vi "Score Particles.vi"(8 "Area Size Limit":i32=444, 9 "Particle Count Limit":i32=10, 11 "Image Refnum in":T1) -> (0 "Circle Info":cluster{dbl, dbl, dbl}[](array[cluster]), 2 "Scored Particle Info":T2(array[cluster]), 3 "Image Refnum out":T1)   [LabVIEW 2012]
doc: "Score the largest particles in the image to determine how well they match the target attributes. Specifically, calculate how rectangular a particle is, inspect its aspect ratio, and determine if it is hollow (having pixels on around the edges, but off in the large center)."
uses:
  <vilib>/vision/Image Controls.llb/IMAQ Image.ctl
  <vilib>/vision/NI_Vision_Development_Module.lvlib
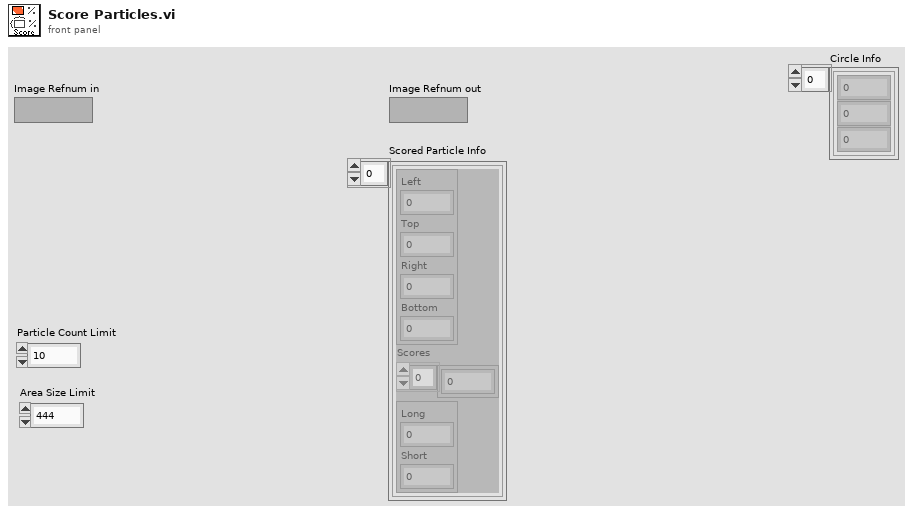
[diagram p1: front panel]
types:
  T1 = typedef "IMAQ Image.ctl" = refnum<image>
  T2 = cluster{cluster{"Left":dbl, "Top":dbl, "Right":dbl, "Bottom":dbl}, "Scores":dbl[], cluster{"Long":dbl, "Short":dbl}}[]
  T3 = typedef "Particle Parameters" = i32
  T4 = typedef "Image Type" = u32
  T5 = cluster{"Left":dbl, "Top":dbl, "Right":dbl, "Bottom":dbl}
  T6 = cluster{cluster{"Left":dbl, "Top":dbl, "Right":dbl, "Bottom":dbl}, dbl[], cluster{"Numeric":dbl, "Numeric":dbl}}
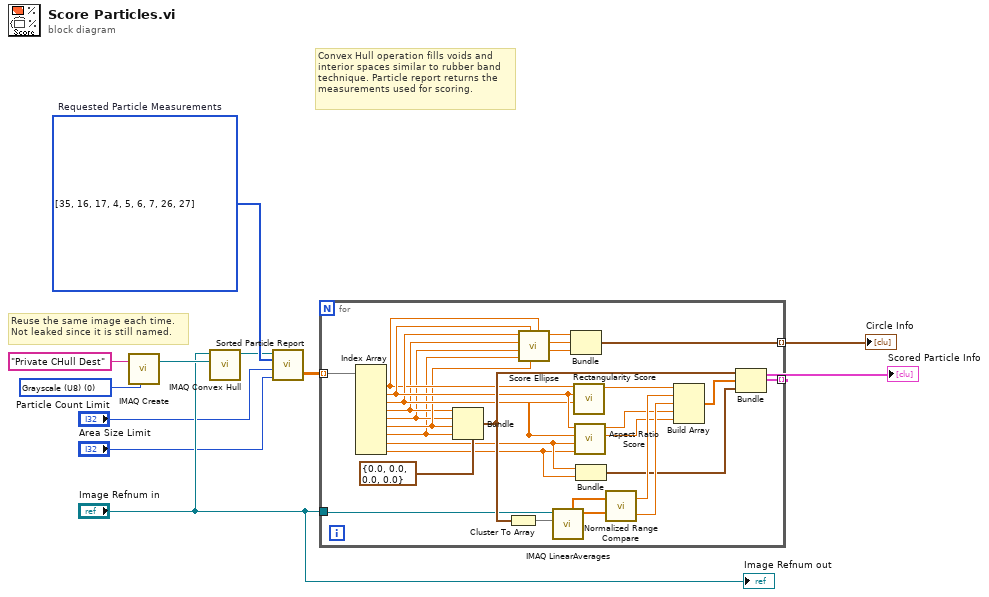
[diagram p0: block diagram]
diagram:
  w3 = T3[] [35, 16, 17, 4, 5, 6, 7, 26, 27] items=["Center of Mass X", "Center of Mass Y", "First Pixel X", "First Pixel Y", "Bounding Rect Left", "Bounding Rect Top", "Bounding Rect Right", "Bounding Rect Bottom", "Max Feret Diameter Start X", "Max Feret Diameter Start Y", "Max Feret Diameter End X", "Max Feret Diameter End Y", "Max Horiz. Segment Length Left", "Max Horiz. Segment Length Right", "Max Horiz. Segment Length Row", "-", "Bounding Rect Width", "Bounding Rect Height", "Bounding Rect Diagonal", "Perimeter", "Convex Hull Perimeter", "Holes' Perimeter", "Max Feret Diameter", "Equivalent Ellipse Major Axis", "Equivalent Ellipse Minor Axis", "Equivalent Ellipse Minor Axis (Feret)", "Equivalent Rect Long Side", "Equivalent Rect Short Side", "Equivalent Rect Diagonal", "Equivalent Rect Short Side (Feret)", "Average Horiz. Segment Length", "Average Vert. Segment Length", "Hydraulic Radius", "Waddel Disk Diameter", "-", "Area", "Holes' Area", "Particle & Holes' Area", "Convex Hull Area", "Image Area", "-", "Number of Holes", "Number of Horiz. Segments", "Number of Vert. Segments", "-", "Orientation", "Max Feret Diameter Orientation", "-", "% Area/Image Area", "% Area/(Particle & Holes' Area)", "Ratio of Equivalent Ellipse Axes", "Ratio of Equivalent Rect Sides", "-", "Elongation Factor", "Compactness Factor", "Heywood Circularity Factor", "Type Factor", "-", "Sum X", "Sum Y", "Sum XX", "Sum XY", "Sum YY", "Sum XXX", "Sum XXY", "Sum XYY", "Sum YYY", "-", "Moment of Inertia XX", "Moment of Inertia XY", "Moment of Inertia YY", "Moment of Inertia XXX", "Moment of Inertia XXY", "Moment of Inertia XYY", "Moment of Inertia YYY", "Norm. Moment of Inertia XX", "Norm. Moment of Inertia XY", "Norm. Moment of Inertia YY", "Norm. Moment of Inertia XXX", "Norm. Moment of Inertia XXY", "Norm. Moment of Inertia XYY", "Norm. Moment of Inertia YYY", "Hu Moment 1", "Hu Moment 2", "Hu Moment 3", "Hu Moment 4", "Hu Moment 5", "Hu Moment 6", "Hu Moment 7"]  # Requested Particle Measurements
  w8 = T4 0 items=["Grayscale (U8)", "Grayscale (I16)", "Grayscale (SGL)", "Complex (CSG)", "RGB (U32)", "HSL (U32)", "RGB (U64)", "Grayscale (U16)"] ("Image Type")
  # "Reuse the same image each time.\nNot leaked since it is still named."
  # "Convex Hull operation fills voids and\ninterior spaces similar to rubber band\ntechnique. Particle report returns the\nmeasurements used for scoring."
  n1 = call "IMAQ Create"("Image Name"="Private CHull Dest", "Image Type"=w8) -> ("New Image"=w7:T1)  [unwired: 2 in, 2 out]
  n2 = call "IMAQ Convex Hull"("Image Dst"=w7, "Image Src"="Image Refnum in") -> ("Image Dst Out"=w1:T1)  [unwired: 2 in, 7 out]
  n3 = call "Sorted Particle Report.vi"("Area Size Limit"="Area Size Limit", "Particle Count Limit"="Particle Count Limit", "Pixel Measurements"=w3, "Image in"=w1) -> ("Sorted Data"=w10:dbl[][])  [unwired: 1 out]
  n4 = for {
    tunnel: [w38] -> w11 mode=indexing
    tunnel: "Image Refnum in" -> [w34]
    tunnel: w10 -> [w33] mode=indexing
    tunnel: [w15] -> w2 mode=indexing
    n5 = Index Array(array=w33) -> (element #1=w22:dbl, element #2=w24:dbl, element #3=w23:dbl, element #4=w20:dbl, element #5=w19:dbl, element #6=w21:dbl, element #7=w14:dbl, element #8=w27:dbl, element #9=w26:dbl)  [unwired: 9 in]
    n6 = Bundle(cluster=T5 {"Left"=0.0, "Top"=0.0, "Right"=0.0, "Bottom"=0.0}, "Left"=w20, "Top"=w19, "Right"=w21, "Bottom"=w14) -> (w37:T5)
    n7 = Cluster To Array(cluster=w37) -> (array=w35:dbl[])
    n8 = call "Score Ellipse.vi"("Bottom"=w14, "Area"=w22, "Right"=w21, "Height"=w24, "Top"=w19, "Left"=w20, "Width"=w23) -> ("Y"=w16:dbl, "X"=w17:dbl, "Area %"=w18:dbl)  [unwired: 2 in]
    n9 = call "IMAQ LinearAverages"("Optional Rectangle"=w35, "Image Src"=w34) -> ("Y Axis Averages"=w13:sgl[], "X Axis Averages"=w12:sgl[])  [unwired: 2 in, 6 out]
    n10 = Bundle("Area %"=w18, "X"=w17, "Y"=w16) -> (w15:cluster{"Area %":dbl, "X":dbl, "Y":dbl})  [unwired: 1 in]
    n11 = call "Rectangularity Score.vi"("Height"=w23, "Width"=w24, "Area"=w22) -> ("Score"=w36:dbl)  [unwired: 8 in]
    n12 = call "Aspect Ratio Score.vi"("Equivalent Rect Short"=w26, "Equivalent Rect Long"=w27, "Height"=w23, "Width"=w24) -> ("Outer"=w29:dbl, "Middle"=w30:dbl)  [unwired: 6 in]
    n13 = Bundle("Numeric"=w27, "Numeric"=w26) -> (w25:cluster{"Numeric":dbl, "Numeric":dbl})  [unwired: 1 in]
    n14 = call "Normalized Range Compare.vi"("Y Averages"=w13, "X Averages"=w12) -> ("Y Score"=w31:dbl, "X Score"=w32:dbl)
    n15 = Build Array(w36, w32, w31, w30, w29) -> (w28:dbl[])
    n16 = Bundle(w37, w28, w25) -> (w38:T6)  [unwired: 1 in]
  }
  "Scored Particle Info" <- w11
  "Circle Info" <- w2
  "Image Refnum out" <- "Image Refnum in"
